vi "Reporte.vi"(8 "error in (no error)":errorcluster, 9 "Estado":string[](array[string]), 10 "Equipo":string, 11 "Aplicacion in":refnum<class "Aplicacion.lvclass">) -> (0 "error out":errorcluster, 3 "Aplicacion out":refnum<class "Aplicacion.lvclass">)   [LabVIEW 2019, in "Aplicacion.lvclass"]
uses:
  Aplicacion.lvclass
  <vilib>/Utility/NIReport.llb/Report Type.ctl
  <vilib>/addons/_office/excel.llb/Excel Easy Table (str).vi
  <vilib>/Utility/NIReport.llb/NI_report.lvclass
  Base de Datos/SQLiteConnector/SQLiteConnection.lvclass
  <vilib>/Utility/NIReport.llb/NI_ReportGenerationCore.lvlib
  <vilib>/Utility/NIReport.llb/Excel/NI_Excel.lvclass
  Base de Datos/Base de Datos.lvclass
  <vilib>/addons/_office/NI_ReportGenerationToolkit.lvlib
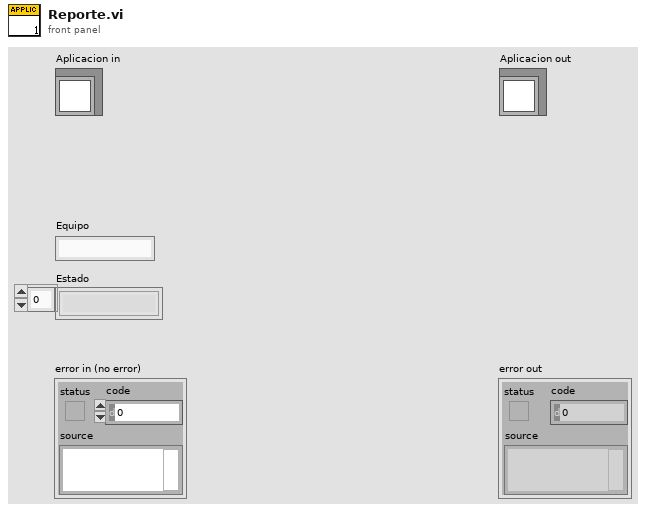
[diagram p1: front panel]
types:
  T1 = typedef "NI_ReportGenerationCore.lvlib/Report Type.ctl" = enum16{"HTML", "Word", "Excel"}
  T2 = enum16{"maximized", "minimized", "normal", "no change"}
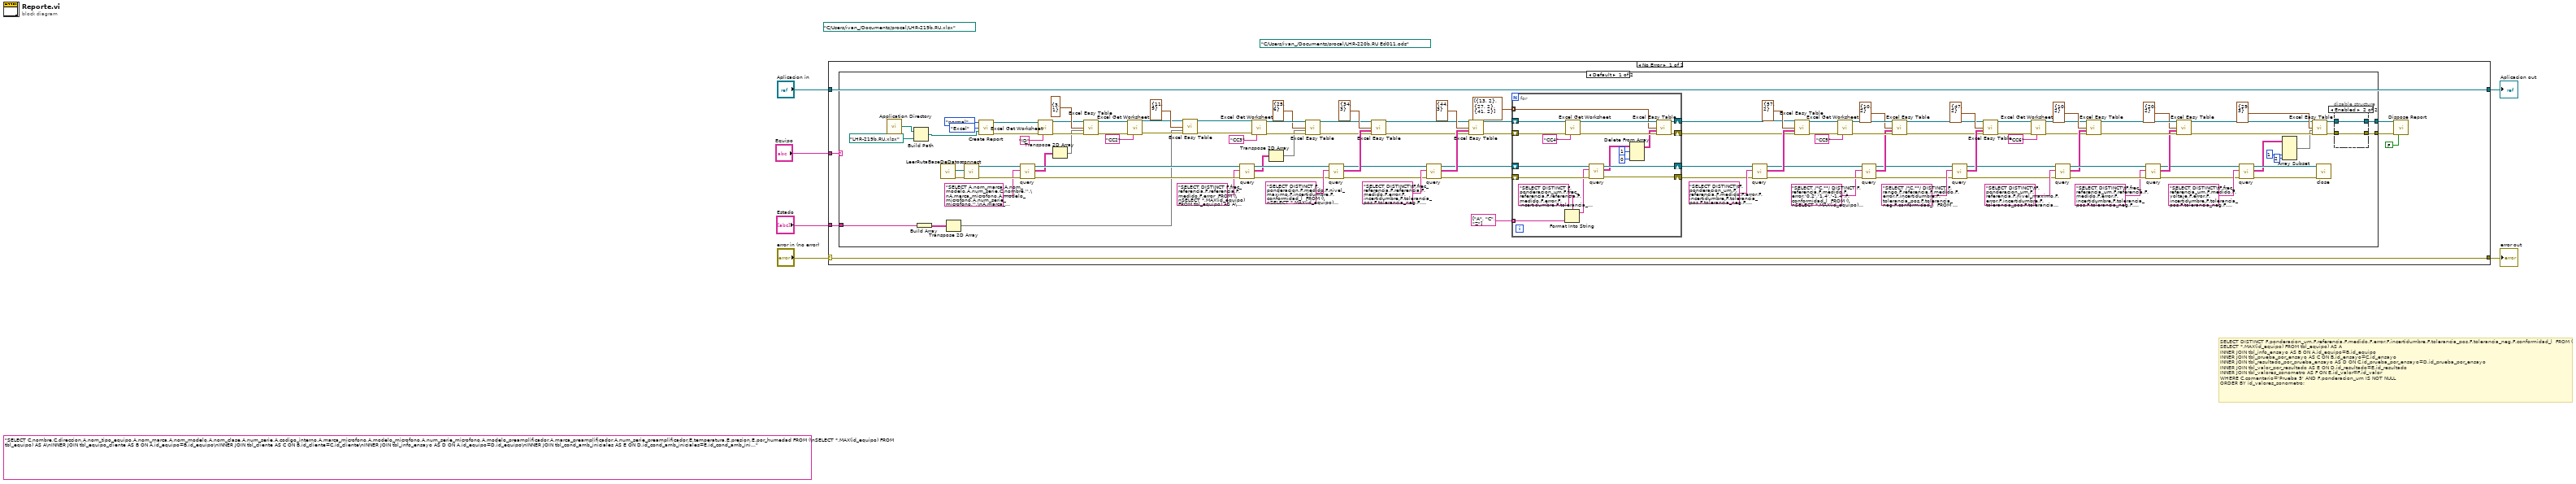
[diagram p0: block diagram]
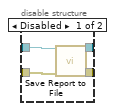
[diagram p2: hidden frame]
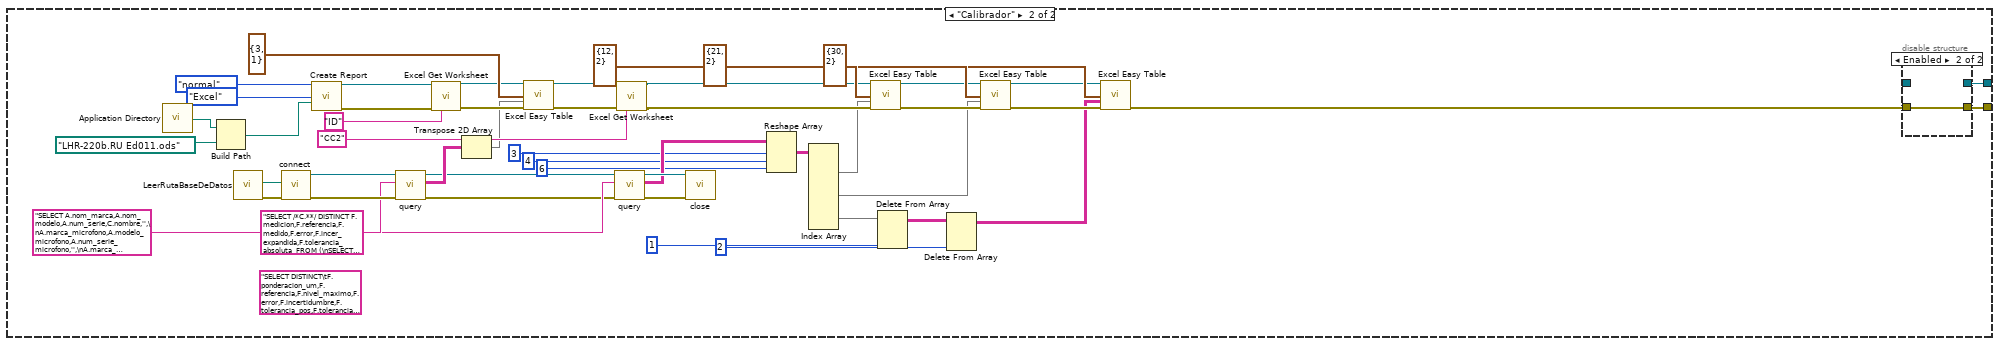
[diagram p3: hidden frame]
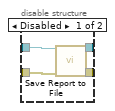
[diagram p4: hidden frame]
diagram:
  (unwired) path "C:/Users/ivan_/Documents/procal/LHR-220b.RU Ed011.ods" ("template (empty)")
  (unwired) path "C:/Users/ivan_/Documents/procal/LHR-219b.RU.xlsx" ("template (empty)")
  (unwired) "SELECT C.nombre,C.direccion,A.nom_tipo_equipo,A.nom_marca,A.nom_modelo,A.nom_clase,A.num_serie,A.codigo_interno,A.marca_microfono,A.modelo_microfono,A.num_serie_microfono,A.modelo_preamplificador,A.marca_preamplificador,A.num_serie_preamplificador,E.temperatura,E.presion,E.por_humedad FROM (\nSELECT *,MAX(id_equipo) FROM tbl_equipo) AS A\nINNER JOIN tbl_equipo_cliente AS B ON A.id_equipo=B.id_equipo\nINNER JOIN tbl_cliente AS C ON B.id_cliente=C.id_cliente\nINNER JOIN tbl_info_ensayo AS D ON A.id_equipo=D.id_equipo\nINNER JOIN tbl_cond_amb_iniciales AS E ON D.id_cond_amb_iniciales=E.id_cond_amb_iniciales;" ("SQL Statement")
  # "SELECT DISTINCT\tF.ponderacion_um,F.referencia,F.medido,F.error,F.incertidumbre,F.tolerancia_pos,F.tolerancia_neg,F.conformidad_l  FROM (\nSELECT *,MAX(id_equipo) FROM tbl_equipo) AS A\nINNER JOIN tbl_info_ensayo AS B ON A.id_equipo=B.id_equipo\nINNER JOIN tbl_prueba_por_ensayo AS C ON B.id_ensayo=C.id_ensayo\nINNER JOIN tbl_resultado_por_prueba_ensayo AS D ON C.id_prueba_por_ensayo=D.id_prueba_por_ensayo\nINNER JOIN tbl_valor_por_resultado AS E ON D.id_resultado=E.id_resultado\nINNER JOIN tbl_valores_sonometro AS F ON E.id_valor=F.id_valor\nWHERE C.comentario='Prueba 5' AND F.ponderacion_um IS NOT NULL\nORDER BY id_valores_sonometro;"
  n1 = case shown="No Error" "error in (no error)" {
    selector: "error in (no error)" -> [w12 w210]
    tunnel: [w12 w210] -> w5
    tunnel: [w13 w209] -> w3
    tunnel: "Aplicacion in" -> [w13 w209]
    tunnel: "Equipo" -> [w8 _]
    tunnel: "Estado" -> [w7 _]
    frame No Error {
      n2 = case shown="Default" w8 {
        tunnel: [w117 w195] -> w11
        tunnel: [w116 w194] -> w10
        tunnel: w7 -> [w19 _]
        frame Default {
          n3 = call <vilib>:"Application Directory.vi"() -> ("Application Directory"=w16:path)
          n4 = Build Path(base path=w16, name or relative path=path "LHR-219b.RU.xlsx" ("template (empty)")) -> (appended path=w14:path)
          n5 = Build Array(w19) -> (w18:string[][])
          n6 = call "LeerRutaBaseDeDatos.vi"() -> ("error out"=w123:errorcluster, "Database Path"=w124:path)  [unwired: 10 in]
          n7 = Transpose 2D Array(2D array=w18) -> (transposed array=w17:string[][])
          n8 = call "connect.vi"("error in (no error)"=w123, "Database Path"=w124) -> ("error out"=w126:errorcluster, "object out"=w125:refnum<class "SQLiteConnection.lvclass">)  [unwired: 8 in]
          n9 = call <vilib>:"Create Report.vi"("window state (normal)"=T2."normal", "report type"=Report_Type."Excel", "template (empty)"=w14) -> ("report out"=w107:refnum<class "NI_report.lvclass">, "error out"=w106:errorcluster)  [unwired: 11 in]
          n10 = call "query.vi"("error in (no error)"=w126, "SQL Statement"="SELECT A.nom_marca,A.nom_modelo,A.num_serie,C.nombre,'',\nA.marca_microfono,A.modelo_microfono,A.num_serie_microfono,'',\nA.marca_preamplificador,A.modelo_preamplificador,A.num_serie_preamplificador,'','',\nA.nom_tipo_equipo,'',A.nom_clase,A.codigo_interno,C.direccion,'','',\n'Medida',E.temperatura,E.presion,E.por_humedad FROM (\nSELECT *,MAX(id_equipo) FROM tbl_equipo\n) AS A\nINNER JOIN tbl_equipo_cliente AS B ON A.id_equipo=B.id_equipo\nINNER JOIN tbl_cliente AS C ON B.id_cliente=C.id_cliente\nINNER JOIN tbl_info_ensayo AS D ON A.id_equipo=D.id_equipo\nINNER JOIN tbl_cond_amb_iniciales AS E ON D.id_cond_amb_iniciales=E.id_cond_amb_iniciales\nORDER BY C.id_cliente DESC\nLIMIT 1", "object in"=w125) -> ("error out"=w128:errorcluster, "result"=w120:string[][], "object out"=w127:refnum<class "SQLiteConnection.lvclass">)  [unwired: 5 in, 1 out]
          n11 = call <vilib>:"Excel Get Worksheet.vi"("report in"=w107, "error in (no error)"=w106, "name (\"\")"="ID" ("name (\"\")")) -> ("report out"=w109:refnum<class "NI_report.lvclass">, "error out"=w110:errorcluster)  [unwired: 11 in]
          n12 = Transpose 2D Array(2D array=w120) -> (transposed array=w105:string[][])
          n13 = call-poly <vilib>:"Excel Easy Table.vi"("report in"=w109, "start (0, 0)"=cluster{"row":i32, "column":i32} {"row"=3, "column"=1}, "text data"=w105, "error in (no error)"=w110) -> ("report out"=w23:refnum<class "NI_report.lvclass">, "error out"=w21:errorcluster)  [unwired: 7 in, 3 out]
          n14 = call <vilib>:"Excel Get Worksheet.vi"("report in"=w23, "error in (no error)"=w21, "name (\"\")"="CC2" ("name (\"\")")) -> ("report out"=w25:refnum<class "NI_report.lvclass">, "error out"=w26:errorcluster)  [unwired: 11 in]
          n15 = call-poly <vilib>:"Excel Easy Table.vi"("report in"=w25, "start (0, 0)"=cluster{"row":i32, "column":i32} {"row"=11, "column"=9}, "text data"=w17, "error in (no error)"=w26) -> ("report out"=w22:refnum<class "NI_report.lvclass">, "error out"=w20:errorcluster)  [unwired: 7 in, 3 out]
          n16 = call "query.vi"("error in (no error)"=w128, "SQL Statement"="SELECT DISTINCT F.frec_referencia,F.referencia,F.medido,F.error  FROM (\nSELECT *,MAX(id_equipo) FROM tbl_equipo) AS A\nINNER JOIN tbl_info_ensayo AS B ON A.id_equipo=B.id_equipo\nINNER JOIN tbl_prueba_por_ensayo AS C ON B.id_ensayo=C.id_ensayo\nINNER JOIN tbl_resultado_por_prueba_ensayo AS D ON C.id_prueba_por_ensayo=D.id_prueba_por_ensayo\nINNER JOIN tbl_valor_por_resultado AS E ON D.id_resultado=E.id_resultado\nINNER JOIN tbl_valores_sonometro AS F ON E.id_valor=F.id_valor\nWHERE C.comentario='Prueba 1'\nORDER BY id_valores_sonometro DESC\nLIMIT 1", "object in"=w127) -> ("error out"=w100:errorcluster, "result"=w99:string[][], "object out"=w101:refnum<class "SQLiteConnection.lvclass">)  [unwired: 5 in, 1 out]
          n17 = call <vilib>:"Excel Get Worksheet.vi"("report in"=w22, "error in (no error)"=w20, "name (\"\")"="CC3" ("name (\"\")")) -> ("report out"=w114:refnum<class "NI_report.lvclass">, "error out"=w113:errorcluster)  [unwired: 11 in]
          n18 = Transpose 2D Array(2D array=w99) -> (transposed array=w98:string[][])
          n19 = call-poly <vilib>:"Excel Easy Table.vi"("report in"=w114, "start (0, 0)"=cluster{"row":i32, "column":i32} {"row"=25, "column"=6}, "text data"=w98, "error in (no error)"=w113) -> ("report out"=w77:refnum<class "NI_report.lvclass">, "error out"=w76:errorcluster)  [unwired: 7 in, 3 out]
          n20 = call "query.vi"("error in (no error)"=w100, "SQL Statement"="SELECT DISTINCT F.ponderacion,F.medido,F.nivel_maximo,F.incertidumbre,F.conformidad_l  FROM (\nSELECT *,MAX(id_equipo) FROM tbl_equipo) AS A\nINNER JOIN tbl_info_ensayo AS B ON A.id_equipo=B.id_equipo\nINNER JOIN tbl_prueba_por_ensayo AS C ON B.id_ensayo=C.id_ensayo\nINNER JOIN tbl_resultado_por_prueba_ensayo AS D ON C.id_prueba_por_ensayo=D.id_prueba_por_ensayo\nINNER JOIN tbl_valor_por_resultado AS E ON D.id_resultado=E.id_resultado\nINNER JOIN tbl_valores_sonometro AS F ON E.id_valor=F.id_valor\nWHERE C.comentario='Prueba 2'\nORDER BY id_valores_sonometro;", "object in"=w101) -> ("error out"=w93:errorcluster, "result"=w103:string[][], "object out"=w94:refnum<class "SQLiteConnection.lvclass">)  [unwired: 5 in, 1 out]
          n21 = call-poly <vilib>:"Excel Easy Table.vi"("report in"=w77, "start (0, 0)"=cluster{"row":i32, "column":i32} {"row"=34, "column"=3}, "text data"=w103, "error in (no error)"=w76) -> ("report out"=w79:refnum<class "NI_report.lvclass">, "error out"=w78:errorcluster)  [unwired: 7 in, 3 out]
          n22 = call "query.vi"("error in (no error)"=w93, "SQL Statement"="SELECT DISTINCT\tF.frec_referencia,F.referencia,F.medido,F.error,F.incertidumbre,F.tolerancia_pos,F.tolerancia_neg,F.conformidad_l  FROM (\nSELECT *,MAX(id_equipo) FROM tbl_equipo) AS A\nINNER JOIN tbl_info_ensayo AS B ON A.id_equipo=B.id_equipo\nINNER JOIN tbl_prueba_por_ensayo AS C ON B.id_ensayo=C.id_ensayo\nINNER JOIN tbl_resultado_por_prueba_ensayo AS D ON C.id_prueba_por_ensayo=D.id_prueba_por_ensayo\nINNER JOIN tbl_valor_por_resultado AS E ON D.id_resultado=E.id_resultado\nINNER JOIN tbl_valores_sonometro AS F ON E.id_valor=F.id_valor\nWHERE C.comentario='Prueba 3'\nORDER BY id_valores_sonometro;", "object in"=w94) -> ("error out"=w89:errorcluster, "result"=w96:string[][], "object out"=w90:refnum<class "SQLiteConnection.lvclass">)  [unwired: 5 in, 1 out]
          n23 = call-poly <vilib>:"Excel Easy Table.vi"("report in"=w79, "start (0, 0)"=cluster{"row":i32, "column":i32} {"row"=44, "column"=3}, "text data"=w96, "error in (no error)"=w78) -> ("report out"=w91:refnum<class "NI_report.lvclass">, "error out"=w92:errorcluster)  [unwired: 7 in, 3 out]
          n24 = for {
            shift-right: [w141] -> w82
            shift-left: w92 -> [w144]
            shift-right: [w142] -> w83
            shift-left: w91 -> [w143]
            shift-right: [w139] -> w81
            shift-left: w90 -> [w140]
            shift-right: [w137] -> w80
            shift-left: w89 -> [w138]
            tunnel: string[] ["A", "C", "Z"] -> [w134] mode=indexing
            tunnel: cluster{"row":i32, "column":i32}[] [{"row"=13, "column"=2}, {"row"=27, "column"=2}, {"row"=41, "column"=2}] -> [w133] mode=indexing
            n25 = Format Into String(format string="SELECT DISTINCT F.ponderacion_um,F.frec_referencia,F.referencia,F.medido,F.error,F.incertidumbre,F.tolerancia_pos,F.tolerancia_neg,F.conformidad_l  FROM (\nSELECT *,MAX(id_equipo) FROM tbl_equipo) AS A\nINNER JOIN tbl_info_ensayo AS B ON A.id_equipo=B.id_equipo\nINNER JOIN tbl_prueba_por_ensayo AS C ON B.id_ensayo=C.id_ensayo\nINNER JOIN tbl_resultado_por_prueba_ensayo AS D ON C.id_prueba_por_ensayo=D.id_prueba_por_ensayo\nINNER JOIN tbl_valor_por_resultado AS E ON D.id_resultado=E.id_resultado\nINNER JOIN tbl_valores_sonometro AS F ON E.id_valor=F.id_valor\nWHERE C.comentario='Prueba 4' AND F.ponderacion_um='%s'\nORDER BY id_valores_sonometro;" ("SQL Statement"), w134) -> (resulting string=w135:string)  [unwired: 2 in, 1 out]
            n26 = call <vilib>:"Excel Get Worksheet.vi"("report in"=w143, "error in (no error)"=w144, "name (\"\")"="CC4" ("name (\"\")")) -> ("report out"=w147:refnum<class "NI_report.lvclass">, "error out"=w145:errorcluster)  [unwired: 11 in]
            n27 = call "query.vi"("error in (no error)"=w138, "SQL Statement"=w135, "object in"=w140) -> ("error out"=w137:errorcluster, "result"=w132:string[][], "object out"=w139:refnum<class "SQLiteConnection.lvclass">)  [unwired: 5 in, 1 out]
            n28 = Delete From Array(array=w132, length=1, index (col)=0 ("disabled index (col)")) -> (array with subset deleted=w131:string[][])  [unwired: 1 in, 1 out]
            n29 = call-poly <vilib>:"Excel Easy Table.vi"("report in"=w147, "start (0, 0)"=w133, "text data"=w131, "error in (no error)"=w145) -> ("report out"=w142:refnum<class "NI_report.lvclass">, "error out"=w141:errorcluster)  [unwired: 7 in, 3 out]
          }
          n30 = call "query.vi"("error in (no error)"=w80, "SQL Statement"="SELECT DISTINCT\tF.ponderacion_um,F.referencia,F.medido,F.error,F.incertidumbre,F.tolerancia_pos,F.tolerancia_neg,F.conformidad_l  FROM (\nSELECT *,MAX(id_equipo) FROM tbl_equipo) AS A\nINNER JOIN tbl_info_ensayo AS B ON A.id_equipo=B.id_equipo\nINNER JOIN tbl_prueba_por_ensayo AS C ON B.id_ensayo=C.id_ensayo\nINNER JOIN tbl_resultado_por_prueba_ensayo AS D ON C.id_prueba_por_ensayo=D.id_prueba_por_ensayo\nINNER JOIN tbl_valor_por_resultado AS E ON D.id_resultado=E.id_resultado\nINNER JOIN tbl_valores_sonometro AS F ON E.id_valor=F.id_valor\nWHERE C.comentario='Prueba 5' AND F.ponderacion_um IS NOT NULL\nORDER BY id_valores_sonometro;", "object in"=w81) -> ("error out"=w71:errorcluster, "result"=w85:string[][], "object out"=w72:refnum<class "SQLiteConnection.lvclass">)  [unwired: 5 in, 1 out]
          n31 = call-poly <vilib>:"Excel Easy Table.vi"("report in"=w83, "start (0, 0)"=cluster{"row":i32, "column":i32} {"row"=57, "column"=2}, "text data"=w85, "error in (no error)"=w82) -> ("report out"=w66:refnum<class "NI_report.lvclass">, "error out"=w67:errorcluster)  [unwired: 7 in, 3 out]
          n32 = call <vilib>:"Excel Get Worksheet.vi"("report in"=w66, "error in (no error)"=w67, "name (\"\")"="CC5" ("name (\"\")")) -> ("report out"=w73:refnum<class "NI_report.lvclass">, "error out"=w75:errorcluster)  [unwired: 11 in]
          n33 = call "query.vi"("error in (no error)"=w71, "SQL Statement"="SELECT /*C.**/ DISTINCT F.referencia,F.medido,F.error,'0.2','1.4','-1.4',F.conformidad_l  FROM (\nSELECT *,MAX(id_equipo) FROM tbl_equipo) AS A\nINNER JOIN tbl_info_ensayo AS B ON A.id_equipo=B.id_equipo\nINNER JOIN tbl_prueba_por_ensayo AS C ON B.id_ensayo=C.id_ensayo\nINNER JOIN tbl_resultado_por_prueba_ensayo AS D ON C.id_prueba_por_ensayo=D.id_prueba_por_ensayo\nINNER JOIN tbl_valor_por_resultado AS E ON D.id_resultado=E.id_resultado\nINNER JOIN tbl_valores_sonometro AS F ON E.id_valor=F.id_valor\nWHERE C.comentario='Prueba 6'\nORDER BY F.id_valores_sonometro", "object in"=w72) -> ("error out"=w59:errorcluster, "result"=w68:string[][], "object out"=w60:refnum<class "SQLiteConnection.lvclass">)  [unwired: 5 in, 1 out]
          n34 = call-poly <vilib>:"Excel Easy Table.vi"("report in"=w73, "start (0, 0)"=cluster{"row":i32, "column":i32} {"row"=10, "column"=2}, "text data"=w68, "error in (no error)"=w75) -> ("report out"=w61:refnum<class "NI_report.lvclass">, "error out"=w62:errorcluster)  [unwired: 7 in, 3 out]
          n35 = call "query.vi"("error in (no error)"=w59, "SQL Statement"="SELECT /*C.**/ DISTINCT F.rango,F.referencia,F.medido,F.error,F.incertidumbre,F.tolerancia_pos,F.tolerancia_neg,F.conformidad_l  FROM (\nSELECT *,MAX(id_equipo) FROM tbl_equipo) AS A\nINNER JOIN tbl_info_ensayo AS B ON A.id_equipo=B.id_equipo\nINNER JOIN tbl_prueba_por_ensayo AS C ON B.id_ensayo=C.id_ensayo\nINNER JOIN tbl_resultado_por_prueba_ensayo AS D ON C.id_prueba_por_ensayo=D.id_prueba_por_ensayo\nINNER JOIN tbl_valor_por_resultado AS E ON D.id_resultado=E.id_resultado\nINNER JOIN tbl_valores_sonometro AS F ON E.id_valor=F.id_valor\nWHERE C.comentario='Prueba 7' AND F.rango NOT IN('--','')\nORDER BY F.id_valores_sonometro", "object in"=w60) -> ("error out"=w44:errorcluster, "result"=w63:string[][], "object out"=w45:refnum<class "SQLiteConnection.lvclass">)  [unwired: 5 in, 1 out]
          n36 = call-poly <vilib>:"Excel Easy Table.vi"("report in"=w61, "start (0, 0)"=cluster{"row":i32, "column":i32} {"row"=47, "column"=2}, "text data"=w63, "error in (no error)"=w62) -> ("report out"=w43:refnum<class "NI_report.lvclass">, "error out"=w42:errorcluster)  [unwired: 7 in, 3 out]
          n37 = call <vilib>:"Excel Get Worksheet.vi"("report in"=w43, "error in (no error)"=w42, "name (\"\")"="CC6" ("name (\"\")")) -> ("report out"=w48:refnum<class "NI_report.lvclass">, "error out"=w46:errorcluster)  [unwired: 11 in]
          n38 = call "query.vi"("error in (no error)"=w44, "SQL Statement"="SELECT DISTINCT\tF.ponderacion_um,F.referencia,F.nivel_maximo,F.error,F.incertidumbre,F.tolerancia_pos,F.tolerancia_neg,F.conformidad_l  FROM (\nSELECT *,MAX(id_equipo) FROM tbl_equipo) AS A\nINNER JOIN tbl_info_ensayo AS B ON A.id_equipo=B.id_equipo\nINNER JOIN tbl_prueba_por_ensayo AS C ON B.id_ensayo=C.id_ensayo\nINNER JOIN tbl_resultado_por_prueba_ensayo AS D ON C.id_prueba_por_ensayo=D.id_prueba_por_ensayo\nINNER JOIN tbl_valor_por_resultado AS E ON D.id_resultado=E.id_resultado\nINNER JOIN tbl_valores_sonometro AS F ON E.id_valor=F.id_valor\nWHERE C.comentario='Prueba 8' AND F.ponderacion_um IS NOT NULL\nORDER BY id_valores_sonometro\nLIMIT 5;", "object in"=w45) -> ("error out"=w58:errorcluster, "result"=w51:string[][], "object out"=w57:refnum<class "SQLiteConnection.lvclass">)  [unwired: 5 in, 1 out]
          n39 = call-poly <vilib>:"Excel Easy Table.vi"("report in"=w48, "start (0, 0)"=cluster{"row":i32, "column":i32} {"row"=10, "column"=2}, "text data"=w51, "error in (no error)"=w46) -> ("report out"=w56:refnum<class "NI_report.lvclass">, "error out"=w55:errorcluster)  [unwired: 7 in, 3 out]
          n40 = call "query.vi"("error in (no error)"=w58, "SQL Statement"="SELECT DISTINCT\tF.frec_referencia_um,F.referencia,F.medido,F.error,F.incertidumbre,F.tolerancia_pos,F.tolerancia_neg,F.conformidad_l  FROM (\nSELECT *,MAX(id_equipo) FROM tbl_equipo) AS A\nINNER JOIN tbl_info_ensayo AS B ON A.id_equipo=B.id_equipo\nINNER JOIN tbl_prueba_por_ensayo AS C ON B.id_ensayo=C.id_ensayo\nINNER JOIN tbl_resultado_por_prueba_ensayo AS D ON C.id_prueba_por_ensayo=D.id_prueba_por_ensayo\nINNER JOIN tbl_valor_por_resultado AS E ON D.id_resultado=E.id_resultado\nINNER JOIN tbl_valores_sonometro AS F ON E.id_valor=F.id_valor\nWHERE C.comentario='Prueba 9'\nORDER BY id_valores_sonometro\nLIMIT 3;", "object in"=w57) -> ("error out"=w38:errorcluster, "result"=w54:string[][], "object out"=w39:refnum<class "SQLiteConnection.lvclass">)  [unwired: 5 in, 1 out]
          n41 = call-poly <vilib>:"Excel Easy Table.vi"("report in"=w56, "start (0, 0)"=cluster{"row":i32, "column":i32} {"row"=20, "column"=2}, "text data"=w54, "error in (no error)"=w55) -> ("report out"=w35:refnum<class "NI_report.lvclass">, "error out"=w34:errorcluster)  [unwired: 7 in, 3 out]
          n42 = call "query.vi"("error in (no error)"=w38, "SQL Statement"="SELECT DISTINCT\tF.frec_referencia_um,F.medido,F.voltaje,F.error,F.incertidumbre,F.tolerancia_pos,F.tolerancia_neg,F.conformidad_l  FROM (\nSELECT *,MAX(id_equipo) FROM tbl_equipo) AS A\nINNER JOIN tbl_info_ensayo AS B ON A.id_equipo=B.id_equipo\nINNER JOIN tbl_prueba_por_ensayo AS C ON B.id_ensayo=C.id_ensayo\nINNER JOIN tbl_resultado_por_prueba_ensayo AS D ON C.id_prueba_por_ensayo=D.id_prueba_por_ensayo\nINNER JOIN tbl_valor_por_resultado AS E ON D.id_resultado=E.id_resultado\nINNER JOIN tbl_valores_sonometro AS F ON E.id_valor=F.id_valor\nWHERE C.comentario='Prueba 10'\nORDER BY id_valores_sonometro\nLIMIT 2;", "object in"=w39) -> ("error out"=w36:errorcluster, "result"=w31:string[][], "object out"=w37:refnum<class "SQLiteConnection.lvclass">)  [unwired: 5 in, 1 out]
          n43 = Array Subset(array=w31, index (col)=1 ("index"), length (col)=2 ("length")) -> (w28:string[][])  [unwired: 2 in]
          n44 = call-poly <vilib>:"Excel Easy Table.vi"("report in"=w35, "start (0, 0)"=cluster{"row":i32, "column":i32} {"row"=29, "column"=3}, "text data"=w28, "error in (no error)"=w34) -> ("report out"=w33:refnum<class "NI_report.lvclass">, "error out"=w32:errorcluster)  [unwired: 7 in, 3 out]
          n45 = call-dynamic "close.vi"("error in (no error)"=w36, "object in"=w37) -> ()  [unwired: 8 in, 2 out]
          n46 = disable-structure shown="Enabled" {
            disable-tunnel: w33 -> [w151 w153]
            disable-tunnel: w32 -> [w150 w152]
            disable-tunnel: [w149 w152] -> w117
            disable-tunnel: [w148 w153] -> w116
            frame Disabled {
              n47 = call-dynamic "Save Report to File.vi"("report in"=w151, "error in (no error)"=w150) -> ("report out"=w148:refnum<class "NI_report.lvclass">, "error out"=w149:errorcluster)  [unwired: 12 in]
            }
            frame Enabled {
            }
          }
        }
        frame "Calibrador" {
          (unwired) "SELECT DISTINCT\tF.ponderacion_um,F.referencia,F.nivel_maximo,F.error,F.incertidumbre,F.tolerancia_pos,F.tolerancia_neg,F.conformidad_l  FROM (\nSELECT *,MAX(id_equipo) FROM tbl_equipo) AS A\nINNER JOIN tbl_info_ensayo AS B ON A.id_equipo=B.id_equipo\nINNER JOIN tbl_prueba_por_ensayo AS C ON B.id_ensayo=C.id_ensayo\nINNER JOIN tbl_resultado_por_prueba_ensayo AS D ON C.id_prueba_por_ensayo=D.id_prueba_por_ensayo\nINNER JOIN tbl_valor_por_resultado AS E ON D.id_resultado=E.id_resultado\nINNER JOIN tbl_valores_sonometro AS F ON E.id_valor=F.id_valor\nWHERE C.comentario='Prueba 8' AND F.ponderacion_um IS NOT NULL\nORDER BY id_valores_sonometro\nLIMIT 5;" ("SQL Statement")
          n48 = call <vilib>:"Application Directory.vi"() -> ("Application Directory"=w156:path)
          n49 = Build Path(base path=w156, name or relative path=path "LHR-220b.RU Ed011.ods" ("template (empty)")) -> (appended path=w154:path)
          n50 = call "LeerRutaBaseDeDatos.vi"() -> ("error out"=w200:errorcluster, "Database Path"=w201:path)  [unwired: 10 in]
          n51 = call "connect.vi"("error in (no error)"=w200, "Database Path"=w201) -> ("error out"=w203:errorcluster, "object out"=w202:refnum<class "SQLiteConnection.lvclass">)  [unwired: 8 in]
          n52 = call <vilib>:"Create Report.vi"("window state (normal)"=T2."normal", "report type"=Report_Type."Excel", "template (empty)"=w154) -> ("report out"=w188:refnum<class "NI_report.lvclass">, "error out"=w186:errorcluster)  [unwired: 11 in]
          n53 = call "query.vi"("error in (no error)"=w203, "SQL Statement"="SELECT A.nom_marca,A.nom_modelo,A.num_serie,C.nombre,'',\nA.marca_microfono,A.modelo_microfono,A.num_serie_microfono,'',\nA.marca_preamplificador,A.modelo_preamplificador,A.num_serie_preamplificador,'','',\nA.nom_tipo_equipo,'',A.nom_clase,A.codigo_interno,C.direccion,'','',\n'Medida',E.temperatura,E.presion,E.por_humedad FROM (\nSELECT *,MAX(id_equipo) FROM tbl_equipo\n) AS A\nINNER JOIN tbl_equipo_cliente AS B ON A.id_equipo=B.id_equipo\nINNER JOIN tbl_cliente AS C ON B.id_cliente=C.id_cliente\nINNER JOIN tbl_info_ensayo AS D ON A.id_equipo=D.id_equipo\nINNER JOIN tbl_cond_amb_iniciales AS E ON D.id_cond_amb_iniciales=E.id_cond_amb_iniciales\nORDER BY C.id_cliente DESC\nLIMIT 1", "object in"=w202) -> ("error out"=w176:errorcluster, "result"=w198:string[][], "object out"=w177:refnum<class "SQLiteConnection.lvclass">)  [unwired: 5 in, 1 out]
          n54 = call <vilib>:"Excel Get Worksheet.vi"("report in"=w188, "error in (no error)"=w186, "name (\"\")"="ID" ("name (\"\")")) -> ("report out"=w190:refnum<class "NI_report.lvclass">, "error out"=w191:errorcluster)  [unwired: 11 in]
          n55 = Transpose 2D Array(2D array=w198) -> (transposed array=w184:string[][])
          n56 = call-poly <vilib>:"Excel Easy Table.vi"("report in"=w190, "start (0, 0)"=cluster{"row":i32, "column":i32} {"row"=3, "column"=1}, "text data"=w184, "error in (no error)"=w191) -> ("report out"=w187:refnum<class "NI_report.lvclass">, "error out"=w185:errorcluster)  [unwired: 7 in, 3 out]
          n57 = call "query.vi"("error in (no error)"=w176, "SQL Statement"="SELECT /*C.**/ DISTINCT F.medicion,F.referencia,F.medido,F.error,F.incer_expandida,F.tolerancia_absoluta  FROM (\nSELECT *,MAX(id_equipo) FROM tbl_equipo) AS A\nINNER JOIN tbl_info_ensayo AS B ON A.id_equipo=B.id_equipo\nINNER JOIN tbl_prueba_por_ensayo AS C ON B.id_ensayo=C.id_ensayo\nINNER JOIN tbl_resultado_por_prueba_ensayo AS D ON C.id_prueba_por_ensayo=D.id_prueba_por_ensayo\nINNER JOIN tbl_valor_por_resultado AS E ON D.id_resultado=E.id_resultado\nINNER JOIN tbl_valores_calibrador AS F ON E.id_valor=F.id_valor\nWHERE C.comentario='Prueba 1'\nORDER BY F.id_valores_calibrador", "object in"=w177) -> ("error out"=w180:errorcluster, "result"=w175:string[][], "object out"=w181:refnum<class "SQLiteConnection.lvclass">)  [unwired: 5 in, 1 out]
          n58 = call <vilib>:"Excel Get Worksheet.vi"("report in"=w187, "error in (no error)"=w185, "name (\"\")"="CC2" ("name (\"\")")) -> ("report out"=w179:refnum<class "NI_report.lvclass">, "error out"=w178:errorcluster)  [unwired: 11 in]
          n59 = call-dynamic "close.vi"("error in (no error)"=w180, "object in"=w181) -> ()  [unwired: 8 in, 2 out]
          n60 = Reshape Array(w175, 3 ("dimension size"), 4 ("dimension size"), 6 ("dimension size")) -> (w171:string[][][])
          n61 = Index Array(array=w171) -> (element #1=w170:string[][], element #2=w162:string[][], element #3=w161:string[][])  [unwired: 9 in]
          n62 = call-poly <vilib>:"Excel Easy Table.vi"("report in"=w179, "start (0, 0)"=cluster{"row":i32, "column":i32} {"row"=12, "column"=2}, "text data"=w170, "error in (no error)"=w178) -> ("report out"=w164:refnum<class "NI_report.lvclass">, "error out"=w167:errorcluster)  [unwired: 7 in, 3 out]
          n63 = Delete From Array(array=w161, index (col)=1 ("index (row)")) -> (array with subset deleted=w158:string[][])  [unwired: 2 in, 1 out]
          n64 = Delete From Array(array=w158, index (col)=2 ("index (row)")) -> (array with subset deleted=w157:string[][])  [unwired: 2 in, 1 out]
          n65 = call-poly <vilib>:"Excel Easy Table.vi"("report in"=w164, "start (0, 0)"=cluster{"row":i32, "column":i32} {"row"=21, "column"=2}, "text data"=w162, "error in (no error)"=w167) -> ("report out"=w163:refnum<class "NI_report.lvclass">, "error out"=w166:errorcluster)  [unwired: 7 in, 3 out]
          n66 = call-poly <vilib>:"Excel Easy Table.vi"("report in"=w163, "start (0, 0)"=cluster{"row":i32, "column":i32} {"row"=30, "column"=2}, "text data"=w157, "error in (no error)"=w166) -> ("error out"=w165:errorcluster)  [unwired: 7 in, 4 out]
          n67 = disable-structure shown="Enabled" {
            disable-tunnel: _ -> [w207 _]
            disable-tunnel: w165 -> [w206 w208]
            disable-tunnel: [w205 w208] -> w195
            disable-tunnel: [w204 _] -> w194
            frame Disabled {
              n68 = call-dynamic "Save Report to File.vi"("report in"=w207, "error in (no error)"=w206) -> ("report out"=w204:refnum<class "NI_report.lvclass">, "error out"=w205:errorcluster)  [unwired: 12 in]
            }
            frame Enabled {
            }
          }
        }
      }
      n69 = call-dynamic "Dispose Report.vi"("report in"=w10, "error in (no error)"=w11, "close report? (T)"=FALSE) -> ()  [unwired: 12 in, 1 out]
    }
    frame Error {
    }
  }
  "error out" <- w5
  "Aplicacion out" <- w3
